vi "Check for Error.vi"(10 "DLL-call return value":u8, 11 "error in (no error)":errorcluster) -> (3 "error out":errorcluster)   [LabVIEW 2022 SP3, in "Logitech Devices.lvlib"]
uses:
  Logitech Devices.lvlib
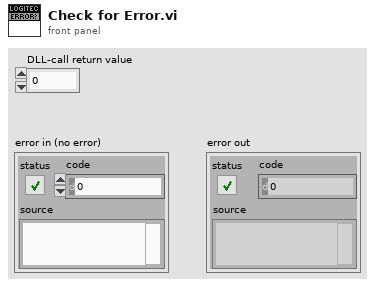
[diagram p1: front panel]
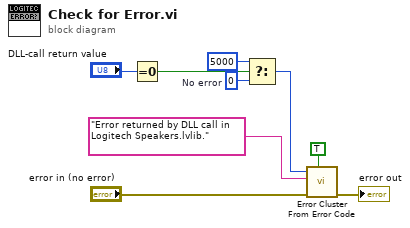
[diagram p0: block diagram]
diagram:
  w5 = 0  # No error
  n1 = Equal To 0?(x="DLL-call return value") -> (x = 0?=w8:bool)
  n2 = Select(t=5000 ("error code (0)"), s=w8, f=w5) -> (s? t:f=w3:i32)
  n3 = call <vilib>:"Error Cluster From Error Code.vi"("show call chain? (False)"=TRUE, "error in (no error)"="error in (no error)", "error message (\"\")"="Error returned by DLL call in Logitech Speakers.lvlib." ("format string"), "error code (0)"=w3) -> ("error out"=→"error out":errorcluster)  [unwired: 5 in]
